vi "Read SICK Data.vi"(8 "error in (no error)":errorcluster, 11 "Simulator in":refnum<class "Simulator.lvclass">) -> (0 "error out":errorcluster, 2 "LIDAR Reading":u32[](array[numeric]), 3 "Simulator out":refnum<class "Simulator.lvclass">)   [LabVIEW 2011, in "Simulator.lvclass"]
uses:
  Simulator.lvclass
  Simulator.lvclass/Simulator.ctl
panel:
  out "Array":cluster{dbl, dbl}[](array[cluster])
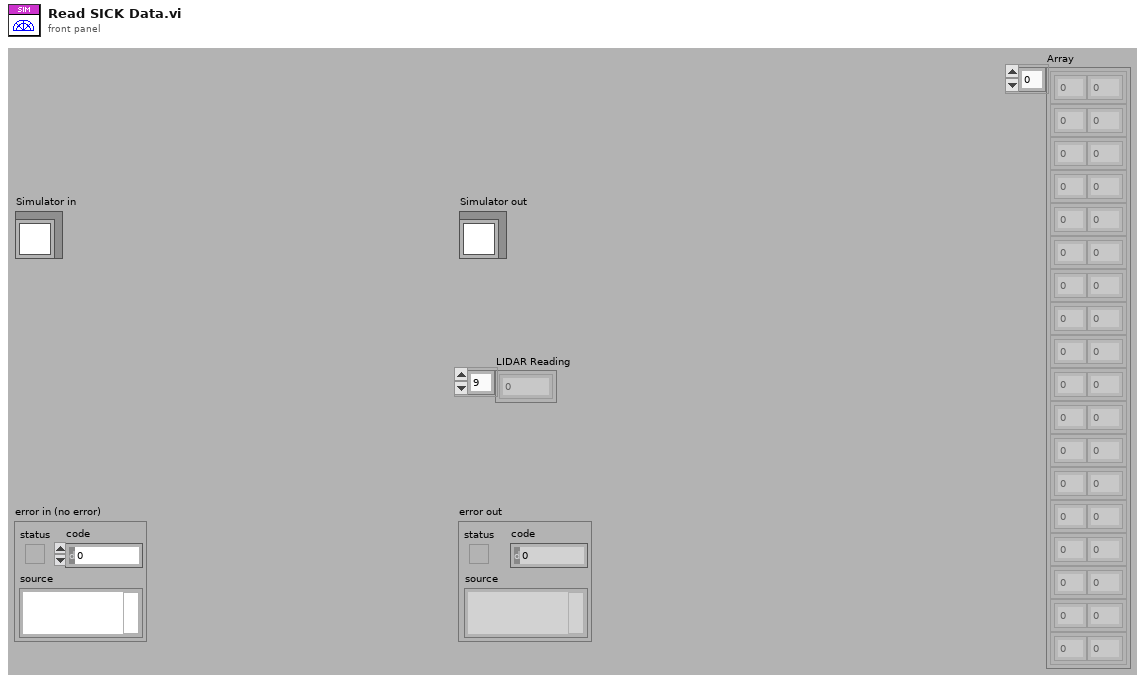
[diagram p1: front panel]
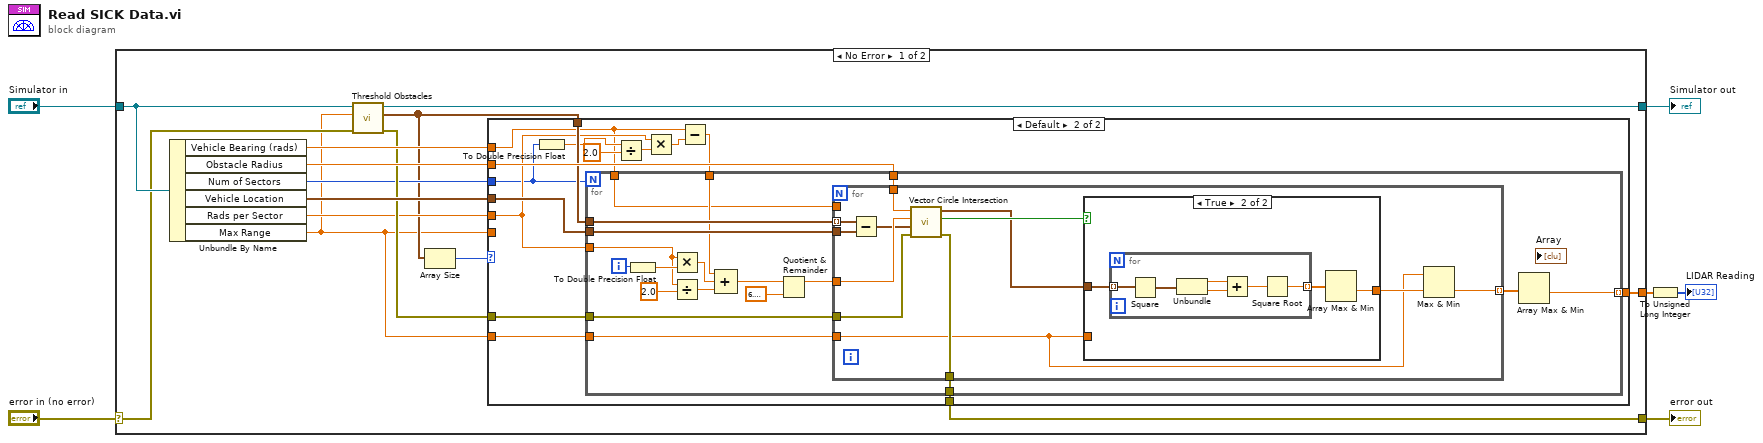
[diagram p0: block diagram]
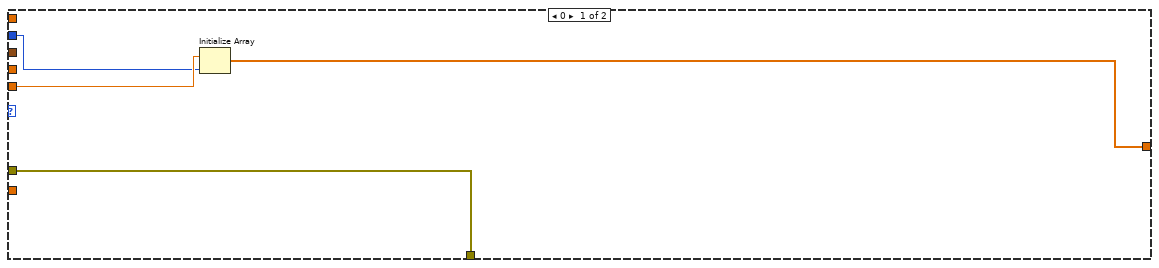
[diagram p2: hidden frame]
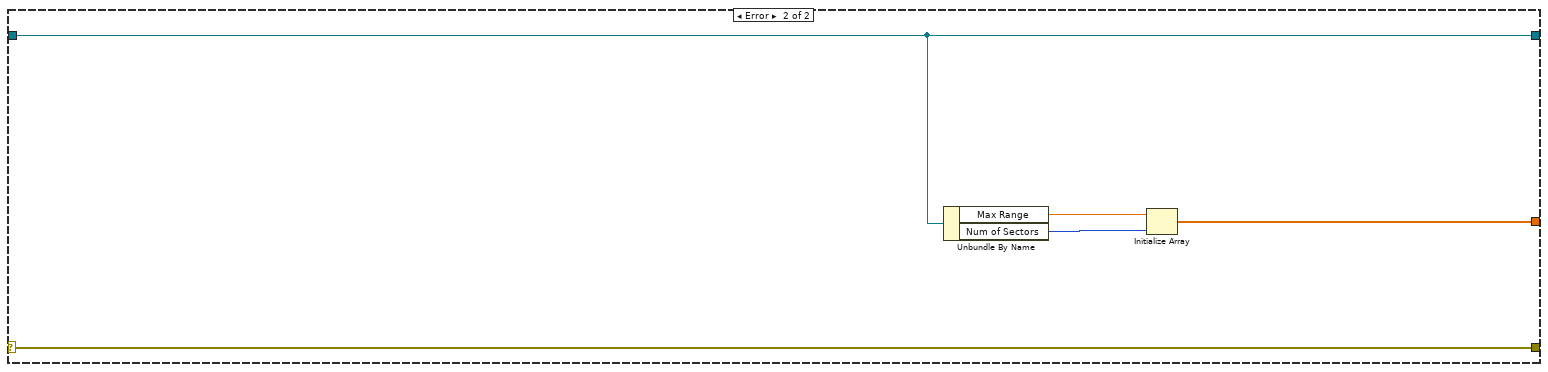
[diagram p4: hidden frame]
diagram:
  n1 = case shown="No Error" "error in (no error)" {
    selector: "error in (no error)" -> [w13 w85]
    tunnel: [w19 w85] -> w5
    tunnel: [w12 w84] -> w3
    tunnel: "Simulator in" -> [w15 w84]
    tunnel: [w17 w81] -> w2
    frame No Error {
      n2 = Unbundle By Name(w15) -> ("Vehicle Bearing (rads)"=w16:dbl, "Obstacle Radius"=w20:dbl, "Num of Sectors"=w10:i32, "Vehicle Location"=w18:cluster{"x":dbl, "y":dbl}, "Rads per Sector"=w11:dbl, "Max Range"=w7:dbl)
      n3 = call-dynamic "Threshold Obstacles.vi"("error in (no error)"=w13, "Threshold"=w7, "Simulator in"=w15) -> ("error out"=w14:errorcluster, "Obstacles Within Threshold"=w8:cluster{"x":dbl, "y":dbl}[], "Simulator out"=w12:refnum<class "Simulator.lvclass">)  [unwired: 6 in]
      n4 = Array Size(array=w8) -> (size(s)=w9:i32)
      n5 = case shown="Default" w9 {
        tunnel: w20 -> [_ w39]
        tunnel: [w24 w38] -> w19
        tunnel: w18 -> [_ w37]
        tunnel: [w23 w36] -> w17
        tunnel: w16 -> [_ w25]
        tunnel: w8 -> [_ w35]
        tunnel: w14 -> [w24 w34]
        tunnel: w7 -> [_ w33]
        tunnel: w11 -> [_ w29]
        tunnel: w10 -> [w21 w27]
        tunnel: w7 -> [w22 _]
        frame 0 {
          n6 = Initialize Array(w22, w21) -> (w23:dbl[])
        }
        frame Default {
          n7 = To Double Precision Float(number=w27) -> (double precision float=w28:dbl)
          n8 = Divide(x=w28, y=2.0) -> (x/y=w30:dbl)
          n9 = Multiply(x=w29, y=w30) -> (x*y=w26:dbl)
          n10 = Subtract(x=w25, y=w26) -> (x-y=w32:dbl)
          n11 = for {
            N: w27 -> [_]
            tunnel: w35 -> [w58]
            tunnel: w37 -> [w57]
            tunnel: w39 -> [w56]
            tunnel: w34 -> [w55]
            tunnel: w29 -> [w45]
            tunnel: [w54] -> w38
            tunnel: w33 -> [w53]
            tunnel: [w51] -> w36 mode=indexing
            tunnel: w32 -> [w44]
            tunnel: w25 -> [w43]
            i -> [w46]
            n12 = To Double Precision Float(number=w46) -> (double precision float=w47:dbl)
            n13 = Multiply(x=w45, y=w47) -> (x*y=w48:dbl)
            n14 = Divide(x=w45, y=2.0) -> (x/y=w50:dbl)
            n15 = Compound Arithmetic op=ADD(w44, w48, w50) -> (w42:dbl)
            n16 = Quotient & Remainder(x=w42, y=6.283185307179586) -> (x-y*floor(x/y)=w41:dbl)  [unwired: 1 out]
            n17 = for {
              tunnel: w58 -> [w66] mode=indexing
              tunnel: w57 -> [w70]
              tunnel: w56 -> [w69]
              tunnel: w55 -> [w68]
              tunnel: [w67] -> w54
              tunnel: w53 -> [w59]
              tunnel: [w60] -> w52 mode=indexing
              tunnel: w41 -> [w65]
              tunnel: w43 -> [_]
              n18 = Subtract(x=w66, y=w70) -> (x-y=w64:cluster{"x":dbl, "y":dbl})
              n19 = call "Vector Circle Intersection.vi"("error in (no error)"=w68, "Circle Center"=w64, "Vector Bearing"=w65, "Circle Radius"=w69) -> ("error out"=w67:errorcluster, "Intersection?"=w63:bool, "Points of Intersection"=w62:cluster{dbl, dbl}[])  [unwired: 5 in]
              n20 = case shown="True" w63 {
                tunnel: w62 -> [_ w74]
                tunnel: w59 -> [w71 _]
                tunnel: [w71 w72] -> w61
                frame False {
                  # "If there was no intersection\nreturn the max range of the\nLIDAR"
                }
                frame True {
                  n21 = for {
                    tunnel: w74 -> [w75] mode=indexing
                    tunnel: [w76] -> w73 mode=indexing
                    n22 = Square(x=w75) -> (x^2=w80:cluster{dbl, dbl})
                    n23 = Unbundle(w80) -> (w78:dbl, w79:dbl)
                    n24 = Add(x=w78, y=w79) -> (x+y=w77:dbl)
                    n25 = Square Root(x=w77) -> (sqrt(x)=w76:dbl)
                  }
                  n26 = Array Max & Min(array=w73) -> (min value=w72:dbl)  [unwired: 3 out]
                }
              }
              n27 = Max & Min(x=w59, y=w61) -> (min(x,y)=w60:dbl)  [unwired: 1 out]
            }
            n28 = Array Max & Min(array=w52) -> (min value=w51:dbl)  [unwired: 3 out]
          }
        }
      }
    }
    frame Error {
      n29 = Unbundle By Name(w84) -> ("Max Range"=w83:dbl, "Num of Sectors"=w82:i32)
      n30 = Initialize Array(w83, w82) -> (w81:dbl[])
    }
  }
  "error out" <- w5
  "Simulator out" <- w3
  n31 = To Unsigned Long Integer(number=w2) -> (unsigned 32bit integer=→"LIDAR Reading":u32[])
